vi "SO55 Create Control Task.vi"(2 "error in":errorcluster, 3 "Output":T1) -> (0 "error out":errorcluster, 1 "task out":refnum<k21>)   [LabVIEW 2012]
uses:
  <vilib>/DAQmx/create/channels.llb/DAQmx Create Channel (AO-Voltage-Basic).vi
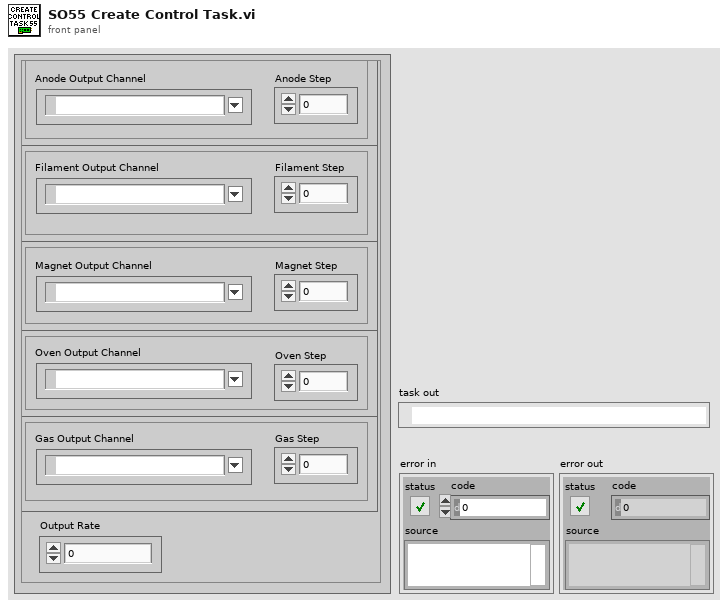
[diagram p1: front panel]
types:
  T1 = cluster{"Anode":cluster{"Anode Output Channel":tag, "Anode Step":dbl}, "Filament":cluster{"Filament Output Channel":tag, "Filament Step":dbl}, "Magnet":cluster{"Magnet Output Channel":tag, "Magnet Step":dbl}, "Oven":cluster{"Oven Output Channel":tag, "Oven Step":dbl}, "Gas":cluster{"Gas Output Channel":tag, "Gas Step":dbl}, "Output Rate":dbl}
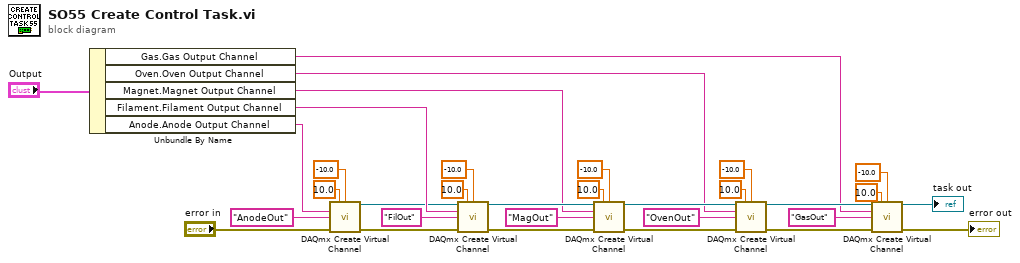
[diagram p0: block diagram]
diagram:
  n1 = Unbundle By Name("Output") -> ("Gas.Gas Output Channel"=w4:tag, "Oven.Oven Output Channel"=w10:tag, "Magnet.Magnet Output Channel"=w16:tag, "Filament.Filament Output Channel"=w23:tag, "Anode.Anode Output Channel"=w31:tag)
  n2 = call-poly <vilib>:"DAQmx Create Virtual Channel.vi"("maximum value"=10.0, "minimum value"=-10.0, "physical channels"=w31, "name to assign"="AnodeOut", "error in"="error in") -> ("task out"=w22:refnum<k21>, "error out"=w24:errorcluster)  [unwired: 9 in]
  n3 = call-poly <vilib>:"DAQmx Create Virtual Channel.vi"("task in"=w22, "maximum value"=10.0, "minimum value"=-10.0, "physical channels"=w23, "name to assign"="FilOut", "error in"=w24) -> ("task out"=w17:refnum<k21>, "error out"=w18:errorcluster)  [unwired: 8 in]
  n4 = call-poly <vilib>:"DAQmx Create Virtual Channel.vi"("task in"=w17, "maximum value"=10.0, "minimum value"=-10.0, "physical channels"=w16, "name to assign"="MagOut", "error in"=w18) -> ("task out"=w11:refnum<k21>, "error out"=w12:errorcluster)  [unwired: 8 in]
  n5 = call-poly <vilib>:"DAQmx Create Virtual Channel.vi"("task in"=w11, "maximum value"=10.0, "minimum value"=-10.0, "physical channels"=w10, "name to assign"="OvenOut", "error in"=w12) -> ("task out"=w5:refnum<k21>, "error out"=w6:errorcluster)  [unwired: 8 in]
  n6 = call-poly <vilib>:"DAQmx Create Virtual Channel.vi"("task in"=w5, "maximum value"=10.0, "minimum value"=-10.0, "physical channels"=w4, "name to assign"="GasOut", "error in"=w6) -> ("task out"=→"task out":refnum<k21>, "error out"=→"error out":errorcluster)  [unwired: 8 in]
